vi "Read Message.vi"(6 "timeout in ms (100)":i32=100, 8 "error in (no error)":errorcluster, 10 "index":i32, 11 "RemoteControl in":refnum<class "RemoteControl.lvclass">) -> (0 "error out":errorcluster, 1 "Data":variant, 2 "Command":string, 3 "RemoteControl out":refnum<class "RemoteControl.lvclass">, 4 "Message ID":i32)   [LabVIEW 2019, in "RemoteControl.lvclass"]
uses:
  RemoteControl.lvclass
  Typedefs/Message--Cluster.ctl
  RemoteControlGlobal.vi
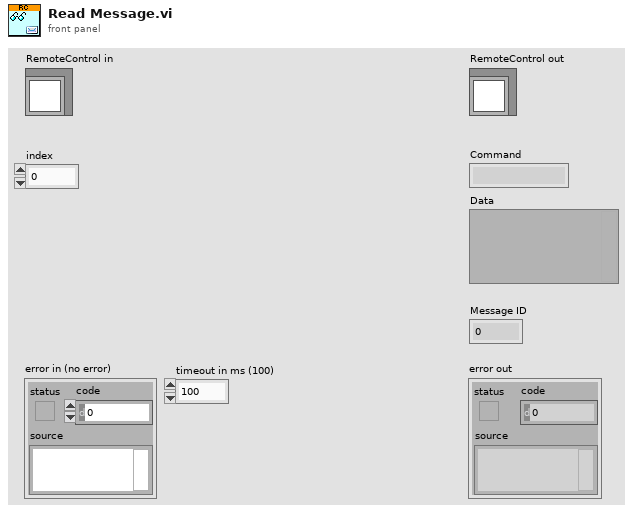
[diagram p1: front panel]
types:
  T1 = typedef "RemoteControl.lvclass/Message--Cluster.ctl" = cluster{"Command":string, "Data":variant, "Message ID":i32}
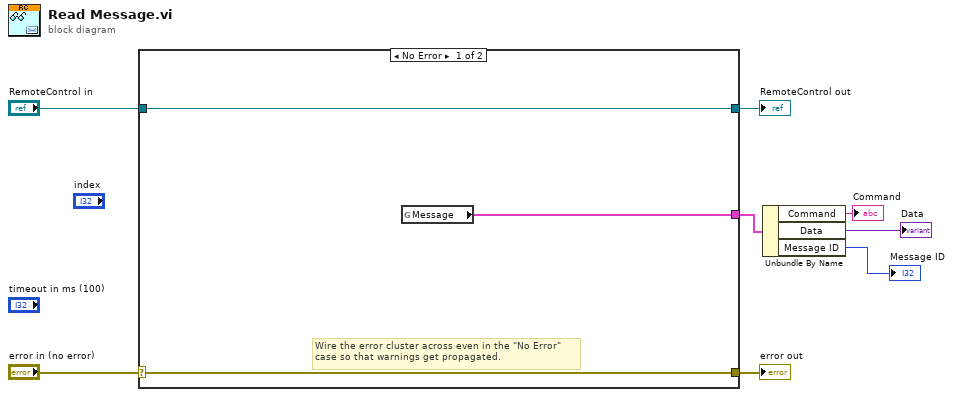
[diagram p0: block diagram]
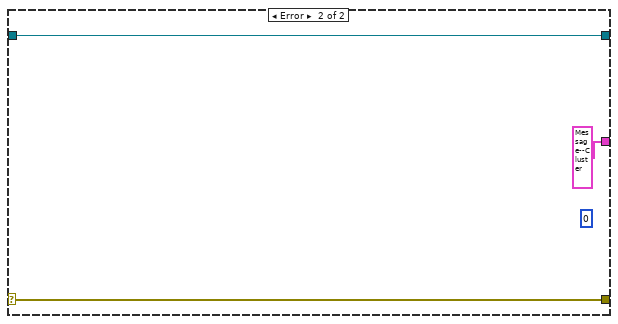
[diagram p2: hidden frame]
diagram:
  n1 = case shown="No Error" "error in (no error)" {
    selector: "error in (no error)" -> [w10 w14]
    tunnel: [w10 w14] -> w7
    tunnel: [w11 w13] -> w5
    tunnel: "RemoteControl in" -> [w11 w13]
    tunnel: [w9 T1 {"Command"="", "Data"=variant, "Message ID"=0} ("Message")] -> w4
    frame No Error {
      # "Wire the error cluster across even in the \"No Error\"\ncase so that warnings get propagated."
      n2 = global read "RemoteControlGlobal.vi" "Message"() -> (w9:T1)
    }
    frame Error {
      (unwired) u32 0 ("Message ID")
    }
  }
  "error out" <- w7
  "RemoteControl out" <- w5
  n3 = Unbundle By Name(w4) -> ("Command"=→"Command":string, "Data"=→"Data":variant, "Message ID"=→"Message ID":i32)
